vi "wiztest.vi"() -> ()   [LabVIEW 2012]
panel:
  out "Numeric Indicator 3":i32
  out "Numeric Indicator 2":i32
  out "Numeric Indicator":i32
  in  "Stop Button":bool
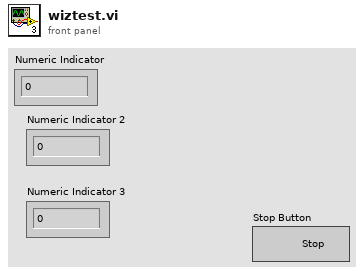
[diagram p1: front panel]
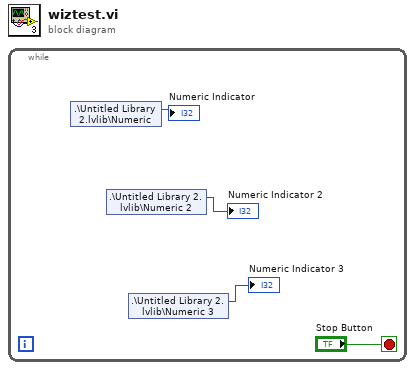
[diagram p0: block diagram]
diagram:
  n1 = while {
    stop <- "Stop Button" stop-if-true
    n2 = shared-variable ".\\Untitled Library 2.lvlib\\Numeric"() -> (→"Numeric Indicator":i32)  [unwired: 1 in, 1 out]
    n3 = shared-variable ".\\Untitled Library 2.lvlib\\Numeric 2"() -> (→"Numeric Indicator 2":i32)  [unwired: 1 in, 1 out]
    n4 = shared-variable ".\\Untitled Library 2.lvlib\\Numeric 3"() -> (→"Numeric Indicator 3":i32)  [unwired: 1 in, 1 out]
  }
